vi "MakeBigTemplate (SubVI).vi"(0 "template image in":u8[][](array[numeric]), 1 "multi image in":i32[][](array[numeric]), 2 "error out":errorcluster) -> (4 "template pic":dbl[][](graph), 5 "smooth template, normalized":dbl[][](graph), 6 "error out 2":errorcluster)   [LabVIEW 2011]
panel:
  out "Best Kernel 2":u8[][](graph)
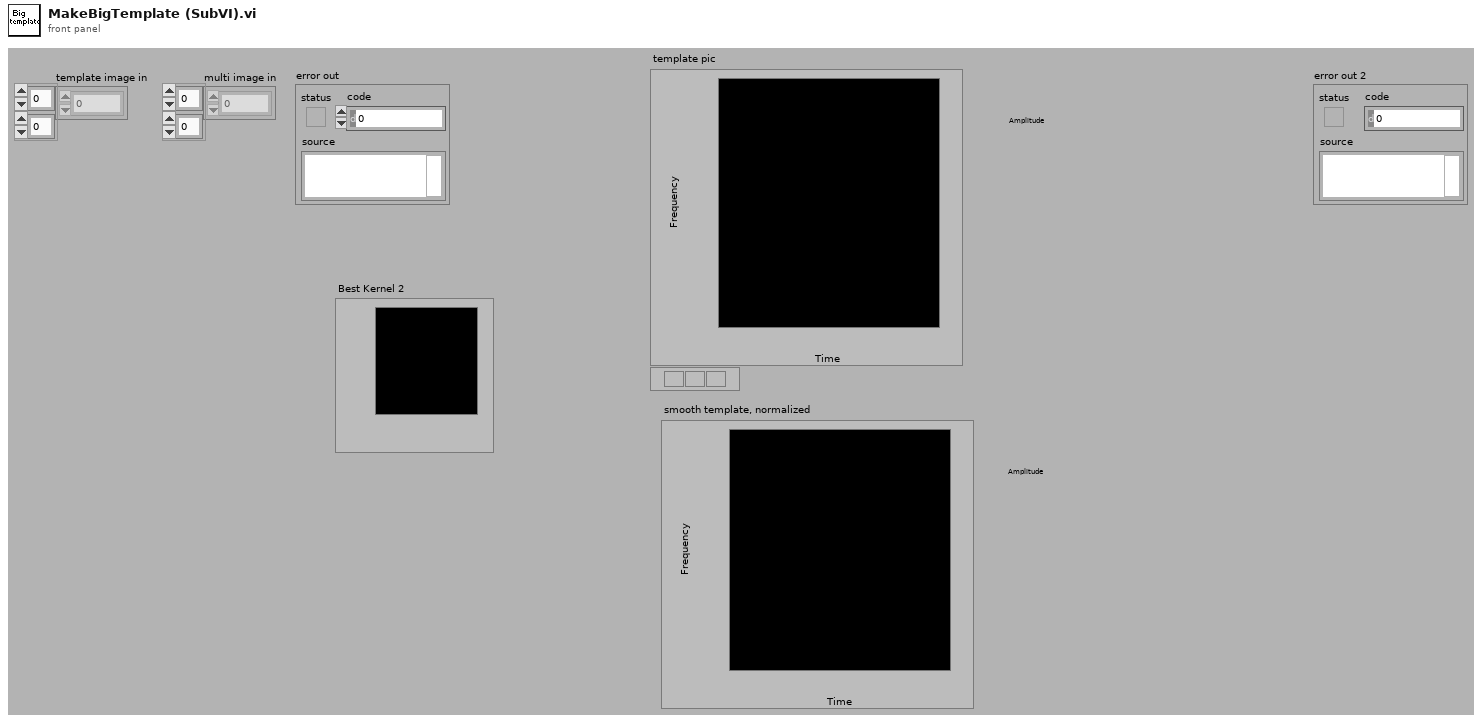
[diagram p1: front panel]
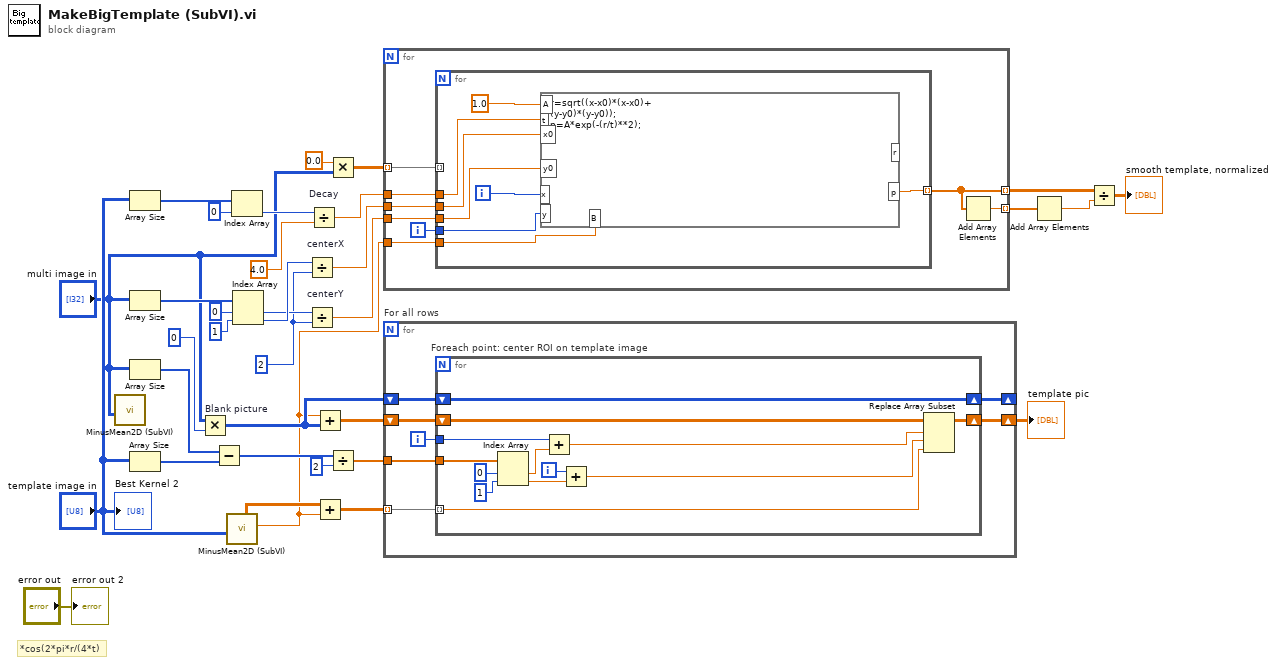
[diagram p0: block diagram]
diagram:
  w22 = 2 ("y")
  # "*cos(2*pi*r/(4*t)"
  n1 = call "MinusMean2D (SubVI).vi"("Image Pixels"="multi image in") -> ()  [unwired: 10 out]
  n2 = Array Size(array="template image in") -> (size(s)=w33:i32[])
  n3 = Array Size(array="multi image in") -> (size(s)=w27:i32[])
  n4 = Array Size(array="multi image in") -> (size(s)=w13:i32[])
  n5 = Array Size(array="template image in") -> (size(s)=w14:i32[])
  n6 = Multiply "Blank picture"(x="multi image in", y=0) -> (x*y=w10:i32[][])
  n7 = Subtract(x=w13, y=w14) -> (x-y=w15:i32[])
  n8 = call "MinusMean2D (SubVI).vi"("Image Pixels"="template image in") -> ("mean"=w6:dbl, "Array"=w12:dbl[][])  [unwired: 8 out]
  n9 = Index Array(array=w33, index=0) -> (element=w31:i32)
  n10 = Index Array(array=w27, index #1=0 ("index"), index #2=1 ("index")) -> (element #1=w23:i32, element #2=w24:i32)
  n11 = Divide "centerX"(x=w24, y=w22) -> (x/y=w21:dbl)
  n12 = Divide "centerY"(x=w23, y=w22) -> (x/y=w20:dbl)
  n13 = Divide "Decay"(x=w31, y=4.0) -> (x/y=w29:dbl)
  n14 = Add(x=w6, y=w10) -> (x+y=w18:dbl[][])
  n15 = Add(x=w12, y=w6) -> (x+y=w11:dbl[][])
  n16 = Multiply(x=0.0, y="multi image in") -> (x*y=w26:dbl[][])
  n17 = Divide(x=w15, y=2) -> (x/y=w17:dbl[])
  n18 = for {
    tunnel: w29 -> [w42]
    tunnel: w26 -> [w41] mode=indexing
    tunnel: w21 -> [w39]
    tunnel: [w36] -> w3 mode=indexing
    tunnel: w20 -> [w38]
    tunnel: w6 -> [w37]
    tunnel: [w35] -> w5 mode=indexing
    i -> [w40]
    n19 = for {
      tunnel: w42 -> [w50]
      tunnel: w41 -> [_] mode=indexing
      tunnel: w40 -> [w47]
      tunnel: w39 -> [w46]
      tunnel: [w45] -> w36 mode=indexing
      tunnel: w38 -> [w44]
      tunnel: w37 -> [w43]
      i -> [w48]
      n20 = formula code="r=sqrt((x-x0)*(x-x0)+\n(y-y0)*(y-y0));\np=A*exp(-(r/t)**2);"("x"=w48, "y"=w47, "t"=w50, "x0"=w46, "A"=1.0 ("input variable"), "y0"=w44, "B"=w43) -> ("p"=w45:dbl)  [unwired: 1 out]
    }
    n21 = Add Array Elements(numeric array=w36) -> (sum=w35:dbl)
  }
  n22 = for "For all rows" {
    tunnel: w17 -> [w57]
    tunnel: w11 -> [w56] mode=indexing
    shift-right: [w54] -> w7
    shift-left: w18 -> [w53]
    shift-right: [w51] -> _
    shift-left: w10 -> [w52]
    i -> [w55]
    n23 = for "Foreach point: center ROI on template image" {
      tunnel: w57 -> [w68]
      tunnel: w56 -> [w59] mode=indexing
      tunnel: w55 -> [w64]
      shift-right: [w60] -> w54
      shift-left: w53 -> [w70]
      shift-right: [w58] -> w51
      shift-left: w52 -> [w58]
      i -> [w69]
      n24 = Index Array(array=w68, index #1=0 ("index"), index #2=1 ("index")) -> (element #1=w63:dbl, element #2=w61:dbl)
      n25 = Add(x=w64, y=w63) -> (x+y=w65:dbl)
      n26 = Add(x=w69, y=w61) -> (x+y=w62:dbl)
      n27 = Replace Array Subset(array=w70, new element=w59, index (row)=w65, index (col)=w62) -> (w60:dbl[][])
    }
  }
  "template pic" <- w7
  n28 = Add Array Elements(numeric array=w5) -> (sum=w4:dbl)
  n29 = Divide(x=w3, y=w4) -> (x/y=→"smooth template, normalized":dbl[][])
  "error out 2" <- "error out"
  "Best Kernel 2" <- "template image in"
